vi "constants.vi"() -> (2 "Resolution Index":i32, 3 "Sampling Frequency [Hz]":dbl)   [LabVIEW 2025, in "LabJackEKG.lvlib"]
uses:
  LabJackEKG.lvlib
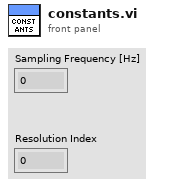
[diagram p1: front panel]
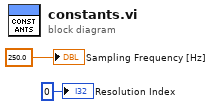
[diagram p0: block diagram]
diagram:
  "Sampling Frequency [Hz]" <- 250.0 ("Sampling Rate [Hz]")
  "Resolution Index" <- 0 ("Resolution Index")
